vi "ConvertEZ-ZONEOutputToWords.vi"(1 "EZ-ZONE Output Cluster":T1={"Loop Control Mode"=10, "Closed Loop Set Point"=75.0, "Open Loop Set Point"=0.0, "Alarm 1 - High Set Point"=150.0, "Alarm 1 - Low Set Point"=0.0, "Alarm 2 - High Set Point"=150.0, "Alarm 2 - Low Set Point"=0.0, "Alarm 3 - High Set Point"=150.0, "Alarm 3 - Low Set Point"=0.0, "Alarm 4 - High Set Point"=150.0, "Alarm 4 - Low Set Point"=0.0, "Profile Action Request"=61, "Profile Start"=0, "Heat Proportional Band"=14.0, "Cool Proportional Band"=14.0, "Time Integral"=180.0, "Time Derivative"=0.0, "Heat Hysteresis"=2.0, "Cool Hysteresis"=2.0, "Dead Band"=0.0} {"Profile Action Request" items=["None"=61, "Start a Profile"=196, "Start a Step"=89, "Pause"=146, "Resume"=147, "End"=148]; "Loop Control Mode" items=["Off"=62, "Auto (closed loop)"=10, "Manual (open loop)"=54]}) -> (0 "Word Array":u32[](array[numeric]))   [LabVIEW 2011]
uses:
  Controls/EZ-ZONE Output Cluster.ctl
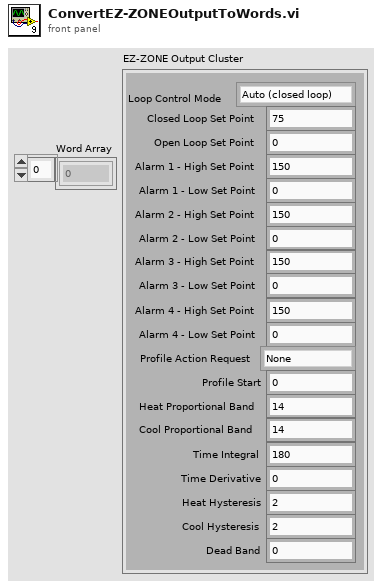
[diagram p1: front panel]
types:
  T1 = typedef "EZ-ZONE Output Cluster.ctl" = cluster{"Loop Control Mode":u32, "Closed Loop Set Point":sgl, "Open Loop Set Point":sgl, "Alarm 1 - High Set Point":sgl, "Alarm 1 - Low Set Point":sgl, "Alarm 2 - High Set Point":sgl, "Alarm 2 - Low Set Point":sgl, "Alarm 3 - High Set Point":sgl, "Alarm 3 - Low Set Point":sgl, "Alarm 4 - High Set Point":sgl, "Alarm 4 - Low Set Point":sgl, "Profile Action Request":u32, "Profile Start":u32, "Heat Proportional Band":sgl, "Cool Proportional Band":sgl, "Time Integral":sgl, "Time Derivative":sgl, "Heat Hysteresis":sgl, "Cool Hysteresis":sgl, "Dead Band":sgl}
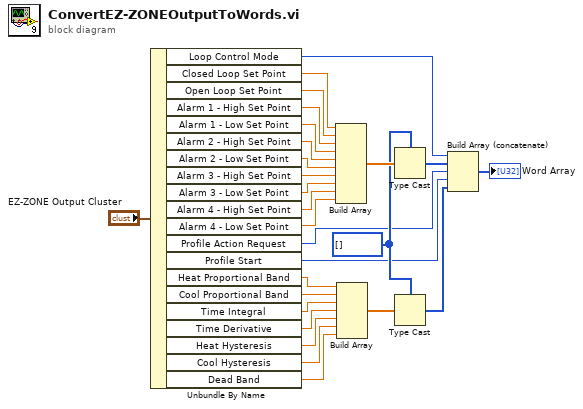
[diagram p0: block diagram]
diagram:
  w7 = u32[] []
  n1 = Unbundle By Name("EZ-ZONE Output Cluster") -> ("Loop Control Mode"=w6:u32, "Closed Loop Set Point"=w26:sgl, "Open Loop Set Point"=w25:sgl, "Alarm 1 - High Set Point"=w24:sgl, "Alarm 1 - Low Set Point"=w23:sgl, "Alarm 2 - High Set Point"=w22:sgl, "Alarm 2 - Low Set Point"=w21:sgl, "Alarm 3 - High Set Point"=w20:sgl, "Alarm 3 - Low Set Point"=w19:sgl, "Alarm 4 - High Set Point"=w18:sgl, "Alarm 4 - Low Set Point"=w17:sgl, "Profile Action Request"=w4:u32, "Profile Start"=w3:u32, "Heat Proportional Band"=w15:sgl, "Cool Proportional Band"=w14:sgl, "Time Integral"=w13:sgl, "Time Derivative"=w12:sgl, "Heat Hysteresis"=w11:sgl, "Cool Hysteresis"=w10:sgl, "Dead Band"=w9:sgl)
  n2 = Build Array(w26, w25, w24, w23, w22, w21, w20, w19, w18, w17) -> (w16:sgl[])
  n3 = Build Array(w15, w14, w13, w12, w11, w10, w9) -> (w8:sgl[])
  n4 = Type Cast(type=w7, x=w16) -> (*(type *) &x=w5:u32[])
  n5 = Type Cast(type=w7, x=w8) -> (*(type *) &x=w2:u32[])
  n6 = Build Array (concatenate)(w6, w5, w4, w3, w2) -> (→"Word Array":u32[])
